vi "Framework.Rx.Async.vi"(8 "error in (no error)":errorcluster, 11 "Framework in":refnum<class "Framework.lvclass">) -> (0 "error out":errorcluster, 3 "Framework out":refnum<class "Framework.lvclass">)   [LabVIEW 2017, in "DSF.Engine.lvlib" / "Framework.lvclass"]
uses:
  Framework.lvclass
  Framework.lvclass/Framework.ctl
  Plugin/Plugin.lvclass/Plugin.ctl
  Timing/DSF.Engine.Timing.lvclass/DSF.Engine.Timing.ctl
  Plugin/Plugin.Get Timing.vi
  Timing/DSF.Engine.Timing.Is Active Cycle.vi
  Timing/DSF.Engine.Timing.Get Decimation.vi
  Timing/DSF.Engine.Timing.Get Offset.vi
  Plugin/Plugin.lvclass
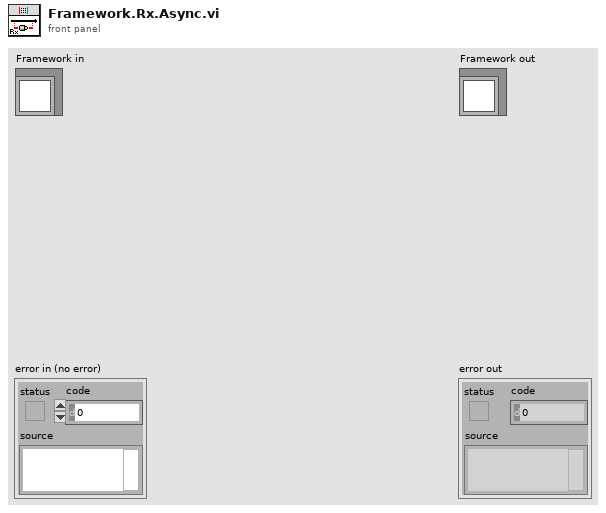
[diagram p1: front panel]
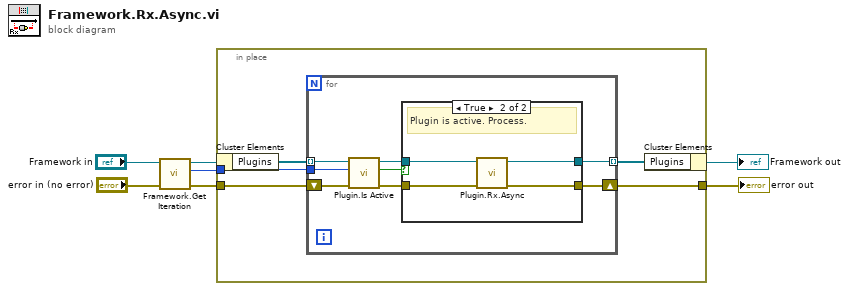
[diagram p0: block diagram]
diagram:
  n1 = call "Framework.Get Iteration.vi"("Framework in"="Framework in") -> ("iteration"=w4:u64, "Framework out"=w1:refnum<class "Framework.lvclass">)  [unwired: 9 in]
  n2 = in-place {
    in-place-border: "error in (no error)" -> [w11]
    in-place-border: [w10] -> w5
    in-place-border: w4 -> [w9]
    n3 = in-place-cluster #1(w1) -> ("Plugins"=w8:refnum<class "Plugin.lvclass">[])
    n4 = for {
      tunnel: w8 -> [w13] mode=indexing
      tunnel: [w18] -> w7 mode=indexing
      shift-right: [w17] -> w10
      shift-left: w11 -> [w16]
      tunnel: w9 -> [w14]
      n5 = call "Plugin.Is Active.vi"("cycle count"=w14, "Plugin in"=w13) -> ("active this cycle?"=w12:bool, "Plugin out"=w15:refnum<class "Plugin.lvclass">)  [unwired: 8 in]
      n6 = case shown="True" w12 {
        tunnel: w15 -> [w20 w24]
        tunnel: [w20 w22] -> w18
        tunnel: [w19 w21] -> w17
        tunnel: w16 -> [w19 w23]
        frame False {
          # "Plugin is not active. Skip."
        }
        frame True {
          # "Plugin is active. Process."
          n7 = call "Plugin.Rx.Async.vi"("error in (no error)"=w23, "Plugin in"=w24) -> ("error out"=w21:errorcluster, "Plugin out"=w22:refnum<class "Plugin.lvclass">)  [unwired: 8 in]
        }
      }
    }
    n8 = in-place-cluster #1("Plugins"=w7) -> (→"Framework out":refnum<class "Framework.lvclass">)
  }
  "error out" <- w5
